vi "Derivative (2D).vi"(8 "error in (no error)":errorcluster, 9 "derivative bin size":dbl=10.0, 10 "Axis Array":dbl[](array[numeric]), 11 "Conductance":dbl[][](graph)) -> (0 "error out":errorcluster, 3 "Transconductance":dbl[][](graph))   [LabVIEW 2016, in "Retrieve and Visualize.lvclass"]
uses:
  Retrieve and Visualize.lvclass
  <userlib>/LevyLab/XY Utilities/subVIs/Append (double array).vi
  <userlib>/LevyLab/XY Utilities/subVIs/Derivative (single).vi
  <userlib>/LevyLab/XY Utilities/xy_utilities.lvlib
panel:
  in  "Type":enum16{"dy/dx vs x", "dx/dy vs y"}(ring)
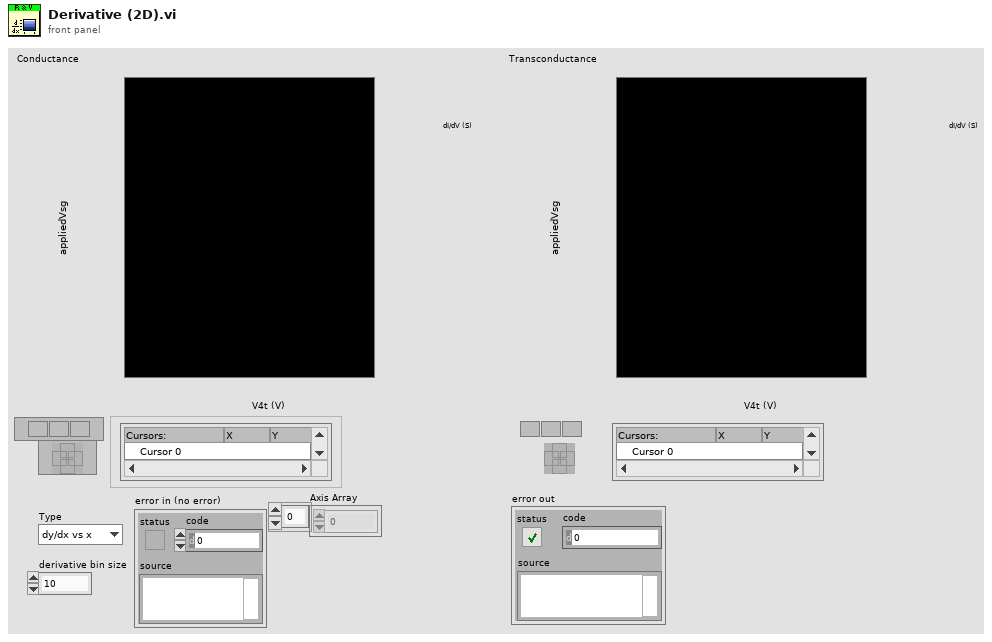
[diagram p1: front panel]
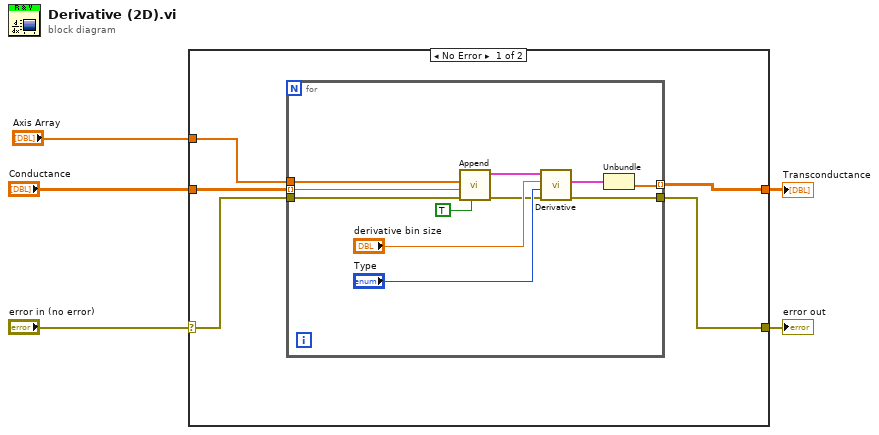
[diagram p0: block diagram]
diagram:
  n1 = case shown="No Error" "error in (no error)" {
    selector: "error in (no error)" -> [w7 w23]
    tunnel: "Axis Array" -> [w10 _]
    tunnel: "Conductance" -> [w9 w22]
    tunnel: [w8 w22] -> w3
    tunnel: [w6 w23] -> w2
    frame No Error {
      n2 = for {
        tunnel: w9 -> [w16] mode=indexing
        tunnel: w10 -> [w17]
        tunnel: [w19] -> w8 mode=indexing
        tunnel: [w12] -> w6
        tunnel: w7 -> [w11]
        n3 = call-poly <userlib>:"Append.vi"("Reset"=TRUE, "error in (no error)"=w11, "Y-array"=w16, "X-array"=w17) -> ("error out"=w13:errorcluster, "XY-data out"=w15:cluster{"X-array":dbl[], "Y-array":dbl[]})  [unwired: 6 in]
        n4 = call-poly <userlib>:"Derivative.vi"("error in (no error)"=w13, "Type"="Type", "Interval (h)"="derivative bin size", "XY-data"=w15) -> ("error out"=w12:errorcluster, "Differential out"=w20:cluster{"X-array":dbl[], "Y-array":dbl[]})  [unwired: 5 in, 1 out]
        n5 = Unbundle(w20) -> ("Y-array"=w19:dbl[])  [unwired: 1 out]
      }
    }
    frame Error {
    }
  }
  "Transconductance" <- w3
  "error out" <- w2
